vi "CRYReport Main.vi"() -> ()   [LabVIEW 2013]
uses:
  CRYReport Global.vi
  CRYWindow/DataView/SubVI/CRYData View Global.vi
  CRYSystem/Data/CRYData & result stacks global.vi
  CRYProject/CRYProject Editor Global.vi
  PrintTxDocDLL.dll
panel:
  in  "ADD_FRAME":bool
  in  "sViewType":string="DataView"
  in  "BtnDATE":bool
  in  "BtnSN":bool
  in  "BtnLot":bool
  in  "BtnOpen":bool
  in  "sInsertVIName":string
  in  "StateOut":bool
  in  "bChange":bool
  in  "BtnPageSize":bool
  in  "sPageSize":string
  in  "BtnPage":bool
  in  "Combo Box":string(combo)
  in  "BtnImage":bool
  in  "BtnPrint":bool
  in  "BtnSave":bool
  in  "TXButtonBar":refnum<k7>(container)
  in  "TXRuler":refnum<k7>(container)
  in  "TXTextControl":refnum<k7>(container)
  in  "stop":bool
  in  "TXStatusBar":refnum<k7>(container)
  in  "bPrintStatus":bool
  in  "bPageStatus":bool
  in  "bStateLoad":bool
  in  "bHitVIS":bool
  in  "InsertVI":bool
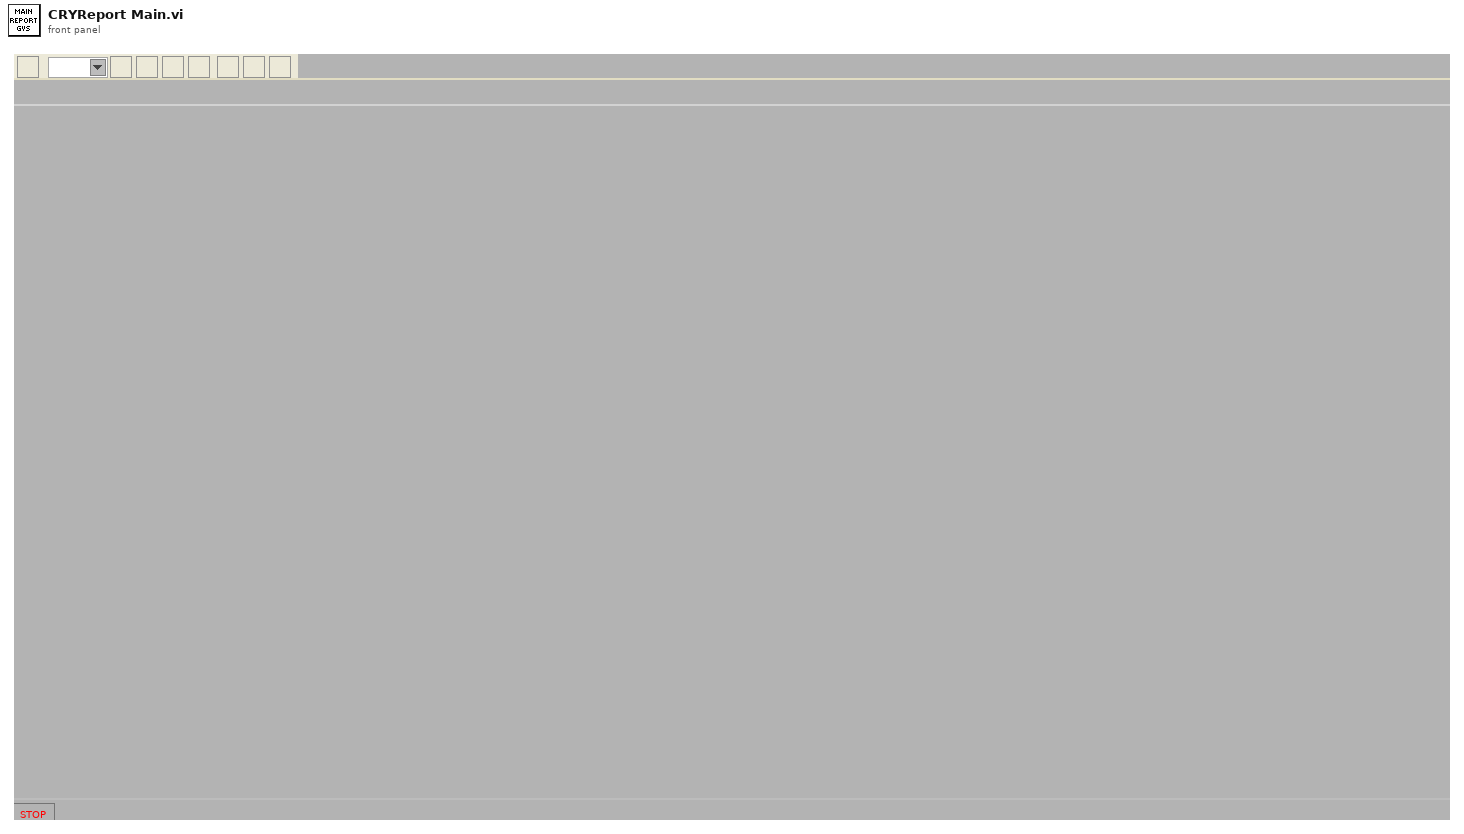
[diagram p1: front panel]
types:
  T1 = cluster{"sAction":string, "sType":string, "sQueueName":string, "sGraphName":string, "sData":string, "nData":i32, "pVIRef":refnum<vi>, "pSPRef":refnum<vi>}
  T2 = enum16{"Left Button", "Center Button", "Right Button", "Window Close"}
  T3 = enum16{"OK", "Yes", "YesNo", "YesNoCancel", "ReplaceAppend"}
  T4 = typedef "CRYDrag Graph.ctl" = cluster{"GraphType":string, "GraphData":variant}
  T5 = typedef "CRYTS.ctl" = cluster{"No.TS":u16, "TS File Path":path, "TS Name":string, "EditStepName":string, "Steps":T6[], "New State":bool, "Change State":bool, "Flattened CurveLib Data":string, "Document Data":string, "EditStepNo":u16, "Operator Start File":string, "Sequence Type":string, "Sequence Language":string}
  T6 = typedef "CRYStep.ctl" = cluster{"No.VI":i32, "Category":string, "StepName":string, "Seq setup flattened":string, "Comment":string, "Steps config.":bool[], "Jump config":i32[], "Start":dbl, "Increment":dbl, "Name":string, "Unit":string, "Y data":u16, "Y prefix":string, "Y dB ref":dbl, "Y unit":string, "Repeat State Array":cluster{"Start":dbl, "Increment":dbl, "Count":i32, "Num":i32}[]}
  T7 = cluster{"nCount":i16, "cFrameList":cluster{"nID":i16, "sName":string, "pVIRef":refnum<vi>, "pSPRef":refnum<vi>, "sTitle":string, "nIDObject":i16, "nIDV":i16, "nWidth":i16, "nHeight":i16, "bImgChange":bool, "sType":string, "sState":string, "sPosition":string, "sData":string}[], "sData":string}
  T8 = cluster{"nID":i16, "sName":string, "pVIRef":refnum<vi>, "pSPRef":refnum<vi>, "sTitle":string, "nIDObject":i16, "nIDV":i16, "nWidth":i16, "nHeight":i16, "bImgChange":bool, "sType":string, "sState":string, "sPosition":string, "sData":string}[]
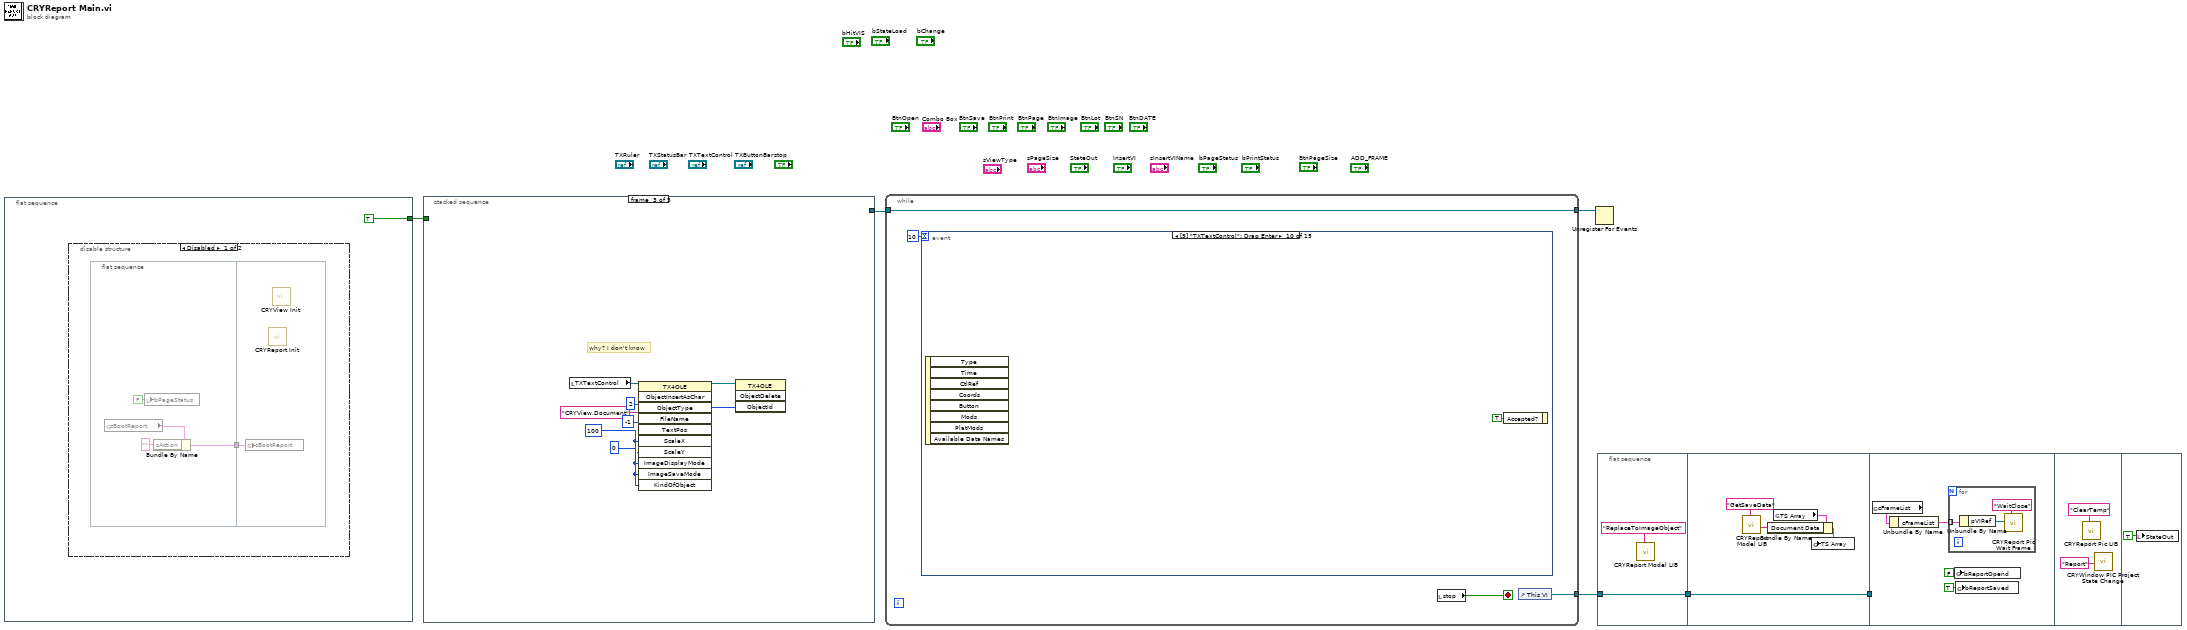
[diagram p0: block diagram]
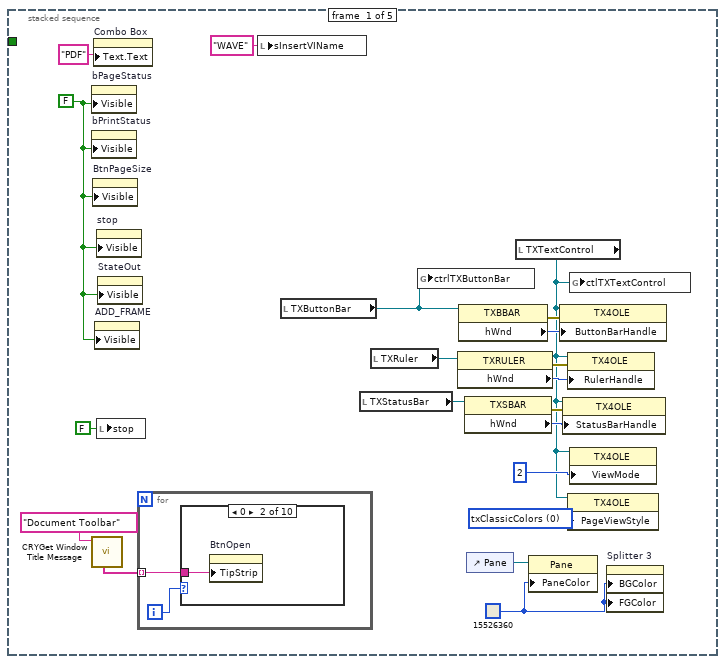
[diagram p3: hidden frame]
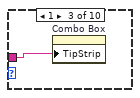
[diagram p5: hidden frame]
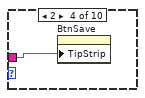
[diagram p6: hidden frame]
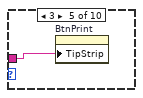
[diagram p7: hidden frame]
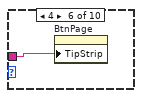
[diagram p8: hidden frame]
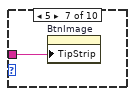
[diagram p9: hidden frame]
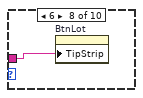
[diagram p10: hidden frame]
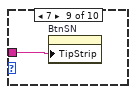
[diagram p11: hidden frame]
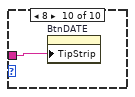
[diagram p12: hidden frame]
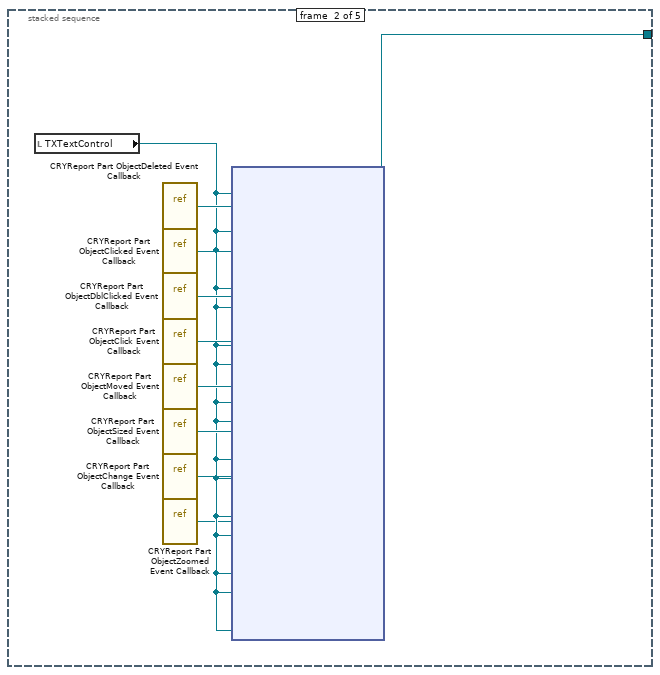
[diagram p13: hidden frame]
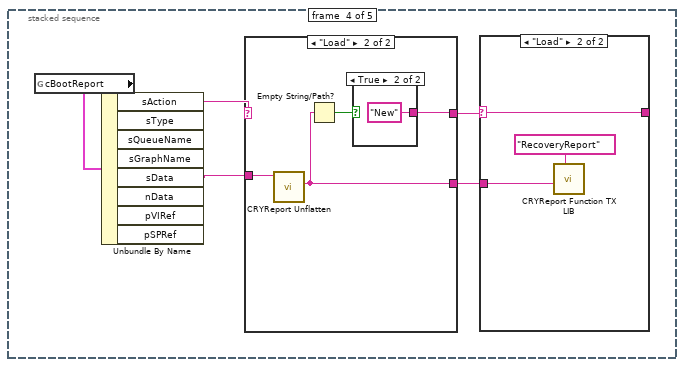
[diagram p14: hidden frame]
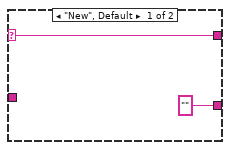
[diagram p16: hidden frame]
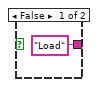
[diagram p17: hidden frame]
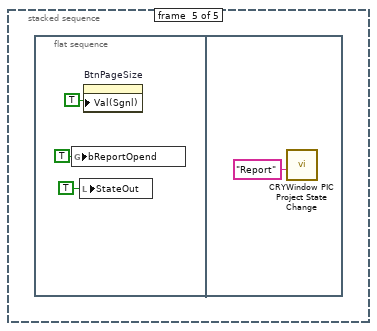
[diagram p18: hidden frame]
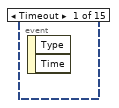
[diagram p19: hidden frame]
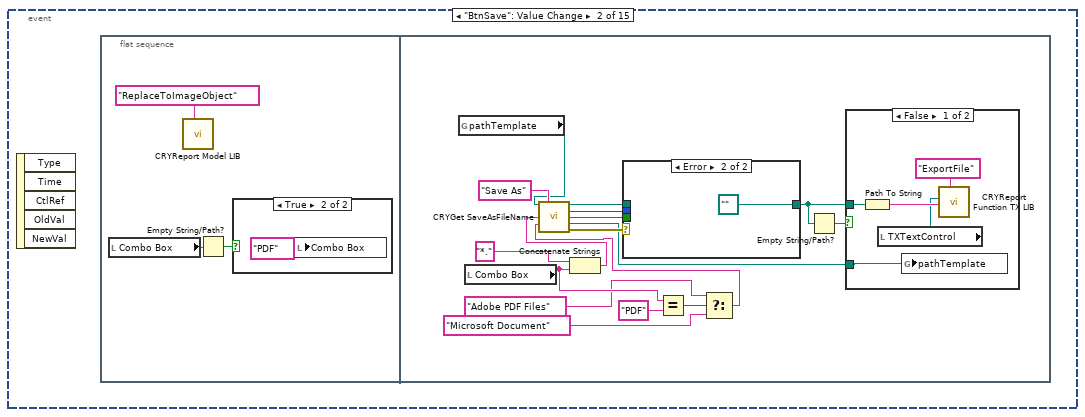
[diagram p20: hidden frame]
diagram:
  n1 = flat-sequence {
    tunnel: [TRUE] -> w3
    frame #0 {
      n2 = disable-structure shown="Disabled" {
        frame Disabled {
          n3 = flat-sequence {
            tunnel: [w9] -> w8
            tunnel: w8 -> [w13]
            frame #0 {
              n4 = global read "CRYReport Global.vi" "cBootReport"() -> (w11:T1)
              n5 = local write "bPageStatus"(FALSE ("bPageStatus")) -> ()
              n6 = Bundle By Name(cluster=w11, "sAction"="") -> (w9:T1)
            }
            frame #1 {
              n7 = global write "CRYReport Global.vi" "cBootReport"(w13) -> ()
              n8 = call "CRYReport Init.vi"() -> ()  [unwired: 12 in]
              n9 = call "CRYView Init.vi"() -> ()  [unwired: 12 in]
            }
          }
        }
        frame Enabled {
        }
      }
    }
  }
  n10 = stacked-sequence {
    tunnel: [_ w45 _ _ _] -> w6
    tunnel: w3 -> [_ _ _ _ _]
    frame #0 {
      w14 = FALSE ("Visible")
      w25 = u32 15526360
      w27 = 0 items=["txClassicColors", "txGradientColors"] ("PageViewStyle")
      n11 = property on="bPageStatus" class="Bool (strict)"("Visible"=w14) -> ()  [unwired: 2 in, 2 out]
      n12 = property on="bPrintStatus" class="Bool (strict)"("Visible"=w14) -> ()  [unwired: 2 in, 2 out]
      n13 = call "CRYGet Window Title Message.vi"("Kind"="Document Toolbar") -> ("Tip Strip"=w15:string[])  [unwired: 5 in, 5 out]
      n14 = property on="BtnPageSize" class="Bool (strict)"("Visible"=w14) -> ()  [unwired: 2 in, 2 out]
      n15 = property on="Combo Box" class="CmbBox"("Text.Text"="PDF") -> ()  [unwired: 2 in, 2 out]
      n16 = property on="ADD_FRAME" class="Bool (strict)"("Visible"=w14) -> ()  [unwired: 2 in, 2 out]
      n17 = property on="stop" class="Bool (strict)"("Visible"=w14) -> ()  [unwired: 2 in, 2 out]
      n18 = local write "stop"(FALSE ("stop")) -> ()
      n19 = property on="StateOut" class="Bool (strict)"("Visible"=w14) -> ()  [unwired: 2 in, 2 out]
      n20 = for {
        tunnel: w15 -> [w35] mode=indexing
        i -> [w34]
        n21 = case shown="0" w34 {
          tunnel: w35 -> [_ w36 w37 w38 w39 w40 w41 w42 w43 w44]
          frame Default {
          }
          frame 0 {
            n22 = property on="BtnOpen" class="Bool (strict)"("TipStrip"=w36) -> ()  [unwired: 2 in, 2 out]
          }
          frame 1 {
            n23 = property on="Combo Box" class="CmbBox"("TipStrip"=w37) -> ()  [unwired: 2 in, 2 out]
          }
          frame 2 {
            n24 = property on="BtnSave" class="Bool (strict)"("TipStrip"=w38) -> ()  [unwired: 2 in, 2 out]
          }
          frame 3 {
            n25 = property on="BtnPrint" class="Bool (strict)"("TipStrip"=w39) -> ()  [unwired: 2 in, 2 out]
          }
          frame 4 {
            n26 = property on="BtnPage" class="Bool (strict)"("TipStrip"=w40) -> ()  [unwired: 2 in, 2 out]
          }
          frame 5 {
            n27 = property on="BtnImage" class="Bool (strict)"("TipStrip"=w41) -> ()  [unwired: 2 in, 2 out]
          }
          frame 6 {
            n28 = property on="BtnLot" class="Bool (strict)"("TipStrip"=w42) -> ()  [unwired: 2 in, 2 out]
          }
          frame 7 {
            n29 = property on="BtnSN" class="Bool (strict)"("TipStrip"=w43) -> ()  [unwired: 2 in, 2 out]
          }
          frame 8 {
            n30 = property on="BtnDATE" class="Bool (strict)"("TipStrip"=w44) -> ()  [unwired: 2 in, 2 out]
          }
        }
      }
      n31 = local write "sInsertVIName"("WAVE" ("sData")) -> ()
      n32 = local read "TXButtonBar"() -> (w17:refnum<k7>)
      n33 = local read "TXStatusBar"() -> (w21:refnum<k7>)
      n34 = local read "TXRuler"() -> (w30:refnum<k7>)
      n35 = global write "CRYReport Global.vi" "ctrlTXButtonBar"(w17) -> ()
      n36 = property class="TXRULER"(reference=w30) -> (error out=w29:errorcluster, "hWnd"=w31:i32)  [unwired: 1 in, 1 out]
      n37 = property class="TXBBAR"(reference=w17) -> (error out=w33:errorcluster, "hWnd"=w32:i32)  [unwired: 1 in, 1 out]
      n38 = property class="TXSBAR"(reference=w21) -> (error out=w22:errorcluster, "hWnd"=w23:i32)  [unwired: 1 in, 1 out]
      n39 = control-ref of="Pane"() -> (w26:refnum<vi>)
      n40 = local read "TXTextControl"() -> (w19:refnum<k7>)
      n41 = property class="Pane"(reference=w26, "PaneColor"=w25) -> ()  [unwired: 1 in, 2 out]
      n42 = property class="TX4OLE"(reference=w19, error in=w33, "ButtonBarHandle"=w32) -> ()  [unwired: 2 out]
      n43 = property class="TX4OLE"(reference=w19, error in=w22, "StatusBarHandle"=w23) -> ()  [unwired: 2 out]
      n44 = property class="TX4OLE"(reference=w19, error in=w29, "RulerHandle"=w31) -> ()  [unwired: 2 out]
      n45 = property class="TX4OLE"(reference=w19, "PageViewStyle"=w27) -> ()  [unwired: 1 in, 2 out]
      n46 = global write "CRYReport Global.vi" "ctlTXTextControl"(w19) -> ()
      n47 = property class="TX4OLE"(reference=w19, "ViewMode"=i16 2) -> ()  [unwired: 1 in, 2 out]
      n48 = property on="Splitter 3" class="Splitter"("BGColor"=w25, "FGColor"=w25) -> ()  [unwired: 2 in, 2 out]
    }
    frame #1 {
      n49 = local read "TXTextControl"() -> (w47:refnum<k7>)
      n50 = vi-ref "CRYReport Part ObjectDeleted Event Callback.vi"() -> ("vi reference"=w54:refnum<vi>)
      n51 = vi-ref "CRYReport Part ObjectClicked Event Callback.vi"() -> ("vi reference"=w52:refnum<vi>)
      n52 = vi-ref "CRYReport Part ObjectDblClicked Event Callback.vi"() -> ("vi reference"=w53:refnum<vi>)
      n53 = vi-ref "CRYReport Part ObjectClick Event Callback.vi"() -> ("vi reference"=w51:refnum<vi>)
      n54 = vi-ref "CRYReport Part ObjectMoved Event Callback.vi"() -> ("vi reference"=w50:refnum<vi>)
      n55 = vi-ref "CRYReport Part ObjectSized Event Callback.vi"() -> ("vi reference"=w49:refnum<vi>)
      n56 = vi-ref "CRYReport Part ObjectChange Event Callback.vi"() -> ("vi reference"=w48:refnum<vi>)
      n57 = vi-ref "CRYReport Part ObjectZoomed Event Callback.vi"() -> ("vi reference"=w46:refnum<vi>)
      n58 = node(w47, w54, w47, w47, w52, w47, w47, w53, w47, w47, w51, w47, w47, w50, w47, w47, w49, w47, w47, w48, w47, w47, w46, w47) -> (w45:refnum<k27>)  [unwired: 2 in, 1 out]
    }
    frame #2 {
      w62 = i16 0 ("ImageDisplayMode")
      w59 = i16 100 ("ScaleX")
      # "why? I don't know"
      n59 = local read "TXTextControl"() -> (w55:refnum<k7>)
      n60 = invoke class="TX4OLE" method="ObjectInsertAsChar"(reference=w55, "ObjectType"=2, "FileName"="CRYView.Document", "TextPos"=-1, "ScaleX"=w59, "ScaleY"=w59, "ImageDisplayMode"=w62, "ImageSaveMode"=w62, "KindOfObject"=w62) -> (reference out=w60:refnum<k7>, "ObjectInsertAsChar"=w61:i16)  [unwired: 2 in, 9 out]
      n61 = invoke class="TX4OLE" method="ObjectDelete"(reference=w60, "ObjectId"=w61) -> ()  [unwired: 2 in, 4 out]
    }
    frame #3 {
      n62 = global read "CRYReport Global.vi" "cBootReport"() -> (w67:T1)
      n63 = Unbundle By Name(w67) -> ("sAction"=w66:string, "sData"=w65:string)  [unwired: 6 out]
      n64 = case shown="\"Load\"" w66 {
        selector: w66 -> [w73 _]
        tunnel: [w73 w75] -> w64
        tunnel: w65 -> [_ w77]
        tunnel: ["" ("Checked Flatten Report") w74] -> w63
        frame "New", Default {
        }
        frame "Load" {
          n65 = call "CRYReport Unflatten.vi"("Flatten Report"=w77) -> ("Checked Flatten Report"=w74:string)  [unwired: 8 in, 2 out]
          n66 = Empty String/Path?(string/path=w74) -> (empty?=w76:bool)
          n67 = case shown="True" w76 {
            tunnel: ["Load" "New"] -> w75
            frame False {
            }
            frame True {
            }
          }
        }
      }
      n68 = case shown="\"Load\"" w64 {
        selector: w64 -> [w68 w71]
        tunnel: [w68 w71] -> _
        tunnel: w63 -> [_ w69]
        frame "New", Default {
        }
        frame "Load" {
          n69 = call "CRYReport Function TX LIB.vi"("sAction"="RecoveryReport", "sData"=w69) -> ()  [unwired: 7 in, 3 out]
        }
      }
    }
    frame #4 {
      n70 = flat-sequence {
        frame #0 {
          n71 = global write "CRYReport Global.vi" "bReportOpend"(TRUE ("bPreportOpend")) -> ()
          n72 = local write "StateOut"(TRUE ("StateOut")) -> ()
          n73 = property on="BtnPageSize" class="Bool (strict)"("Val(Sgnl)"=TRUE ("BtnPageSize")) -> ()  [unwired: 2 in, 2 out]
        }
        frame #1 {
          n74 = call "CRYWindow PIC Project State Change.vi"("sData"="Report") -> ()  [unwired: 11 in]
        }
      }
    }
  }
  n75 = while {
    tunnel: [w87] -> w4
    tunnel: w6 -> [w86]
    tunnel: [w86] -> w5
    stop <- w84 stop-if-true
    n76 = event shown="[9] \"TXTextControl\": Drag Enter" {
      selector: _ -> [_ _ _ _ _ _ _ _ _ _ _ _ _ _ _]
      dyn-events: _ -> [_ _ _ _ _ _ _ _ _ _ _ _ _ _ _]
      timeout: 10 -> [_ _ _ _ _ _ _ _ _ _ _ _ _ _ _]
      event Timeout {
        n77 = event-data() -> ()  [unwired: 1 in, 2 out]
      }
      event "BtnSave": Value Change {
        n78 = event-data() -> ()  [unwired: 1 in, 5 out]
        n79 = flat-sequence {
          frame #0 {
            n80 = local read "Combo Box"() -> (w89:string)
            n81 = call "CRYReport Model LIB.vi"("sAction"="ReplaceToImageObject") -> ()  [unwired: 9 in, 2 out]
            n82 = Empty String/Path?(string/path=w89) -> (empty?=w88:bool)
            n83 = case shown="True" w88 {
              frame False {
              }
              frame True {
                n84 = local write "Combo Box"("PDF" ("Combo Box")) -> ()
              }
            }
          }
          frame #1 {
            n85 = global read "CRYReport Global.vi" "pathTemplate"() -> (w99:path)
            n86 = local read "Combo Box"() -> (w97:string)
            n87 = Concatenate Strings("*." ("string"), w97) -> (w107:string)
            n88 = Equal?(x=w97, y="PDF") -> (x = y?=w95:bool)
            n89 = Select(t="Adobe PDF Files" ("pattern label"), s=w95, f="Microsoft Document" ("pattern label")) -> (s? t:f=w93:string)
            n90 = call "CRYGet SaveAsFileName.vi"("Start path"=w99, "TitleName"="Save As", "pattern (all files)"=w107, "pattern label"=w93) -> ("Path"=w108:path, "Which Button?"=w104:T2, "Is Replace?"=w105:bool, "stripped path"=w98:path, "error out"=w103:errorcluster)  [unwired: 5 in, 2 out]
            n91 = case shown="Error" w103 {
              tunnel: w108 -> [w118 _]
              tunnel: w104 -> [w117 _]
              tunnel: w105 -> [w119 _]
              tunnel: [w114 path "" ("Path")] -> w101
              frame No Error {
                n92 = case shown="True" w119 {
                  tunnel: w118 -> [w122 w124]
                  tunnel: [w122 w124] -> w115
                  tunnel: w117 -> [w123 w125]
                  tunnel: [w123 w125] -> w116
                  frame False {
                  }
                  frame True {
                  }
                }
                n93 = case shown="\"Left Button\", Default" w116 {
                  tunnel: w115 -> [w120 _]
                  tunnel: [w120 path "" ("Path")] -> w114
                  frame "Left Button", Default {
                  }
                  frame "Center Button" {
                  }
                }
              }
              frame Error {
              }
            }
            n94 = Empty String/Path?(string/path=w101) -> (empty?=w100:bool)
            n95 = case shown="False" w100 {
              tunnel: w101 -> [w113 _]
              tunnel: w98 -> [w109 _]
              frame False {
                n96 = Path To String(path=w113) -> (string=w112:string)
                n97 = local read "TXTextControl"() -> (w110:refnum<k7>)
                n98 = global write "CRYReport Global.vi" "pathTemplate"(w109) -> ()
                n99 = call "CRYReport Function TX LIB.vi"("sAction"="ExportFile", "sData"=w112, "TXTextControl"=w110) -> ()  [unwired: 6 in, 3 out]
              }
              frame True {
              }
            }
          }
        }
      }
      event "BtnPageSize": Value Change {
        w139 = 0.5 ("y")
        w142 = 25.4 ("y")
        w145 = 1440.0 ("y")
        n100 = event-data() -> ()  [unwired: 1 in, 5 out]
        n101 = local read "TXTextControl"() -> (w127:refnum<k7>)
        n102 = property class="TX4OLE"(reference=w127) -> ("PageWidth"=w147:i32)  [unwired: 1 in, 2 out]
        n103 = property class="TX4OLE"(reference=w127) -> ("PageHeight"=w146:i32)  [unwired: 1 in, 2 out]
        n104 = Divide(x=w147, y=w145) -> (x/y=w144:dbl)
        n105 = Divide(x=w146, y=w145) -> (x/y=w143:dbl)
        n106 = Multiply(x=w143, y=w142) -> (x*y=w140:dbl)
        n107 = Multiply(x=w144, y=w142) -> (x*y=w141:dbl)
        n108 = Add(x=w141, y=w139) -> (x+y=w136:dbl)
        n109 = Add(x=w140, y=w139) -> (x+y=w135:dbl)
        n110 = Number To Decimal String(number=w136) -> (decimal integer string=w138:string)  [unwired: 1 in]
        n111 = Number To Decimal String(number=w135) -> (decimal integer string=w134:string)  [unwired: 1 in]
        n112 = Concatenate Strings(w138, "*" ("string"), w134) -> (w129:string)
        n113 = case shown="\"148*210\", \"210*148\"" w129 {
          tunnel: ["Custom" "A4" "A3" "A5" "B4" "B5" "Postcard" "Legal" "Tabloid" "Executive" "Screen" "Letter" "Letter Extra" "Letter Plus" "Qurato" "Statement" "SuperA" "SuperB"] -> w131
          frame Default {
          }
          frame "210*297", "297*210" {
          }
          frame "297*420", "420*297" {
          }
          frame "148*210", "210*148" {
          }
          frame "257*364", "364*257" {
          }
          frame "182*257", "257*182" {
          }
          frame "100*147", "147*100" {
          }
          frame "216*356", "356*216" {
          }
          frame "280*432", "432*280" {
          }
          frame "185*267", "267*185" {
          }
          frame "132*166", "166*132" {
          }
          frame "216*280", "280*216" {
          }
          frame "242*305", "305*242" {
          }
          frame "216*323", "323*216" {
          }
          frame "215*275", "275*215" {
          }
          frame "140*216", "216*140" {
          }
          frame "227*356", "356*227" {
          }
          frame "305*487", "487*305" {
          }
        }
        n114 = Concatenate Strings(w131, "(" ("string"), w129, ")" ("string"), "mm" ("string")) -> (w128:string)
        n115 = local write "sPageSize"(w128) -> ()
      }
      event "BtnOpen": Value Change {
        n116 = event-data() -> ()  [unwired: 1 in, 5 out]
        n117 = local read "TXTextControl"() -> (w169:refnum<k7>)
        n118 = invoke class="TX4OLE" method="GetLineCount"(reference=w169) -> ("GetLineCount"=w168:i32)  [unwired: 2 in, 2 out]
        n119 = Greater Than 0?(x=w168) -> ()  [unwired: 1 out]
        n120 = case shown="False" FALSE {
          tunnel: [T2."Left Button" ("Which Button?") w171] -> w167
          frame False {
          }
          frame True {
            n121 = call <vilib>:"Three Button Dialog.vi"("message"="Do you want replace document ?") -> ("Which Button?"=w171:T2)  [unwired: 10 in]
          }
        }
        n122 = case shown="\"Left Button\"" w167 {
          frame "Left Button" {
            n123 = flat-sequence {
              frame #0 {
                n124 = call "CRYReport Model LIB.vi"("sAction"="ReplaceToImageObject") -> ()  [unwired: 9 in, 2 out]
              }
              frame #1 {
                n125 = global read "CRYReport Global.vi" "pathTemplate"() -> (w176:path)
                n126 = call "CRYGet LoadFileName.vi"("pattern label"="Microsoft Document", "pattern (all files)"="*.doc" ("string"), "TitleName"="Open As", "Category Name"="doc" ("string"), "Start path"=w176) -> ("error out"=w180:errorcluster, "stripped path"=w175:path, "Which Button?"=w181:T2, "Path"=w182:path)  [unwired: 3 in]
                n127 = case shown="No Error" w180 {
                  tunnel: w182 -> [w184 _]
                  tunnel: w181 -> [w185 _]
                  tunnel: w175 -> [w183 _]
                  frame No Error {
                    n128 = case shown="\"Center Button\", Default" w185 {
                      tunnel: w184 -> [w190 _]
                      tunnel: w183 -> [w186 _]
                      frame "Left Button" {
                        n129 = Path To String(path=w190) -> (string=w189:string)
                        n130 = local read "TXTextControl"() -> (w187:refnum<k7>)
                        n131 = global write "CRYReport Global.vi" "pathTemplate"(w186) -> ()
                        n132 = call "CRYReport Function TX LIB.vi"("sAction"="OpenFile", "sData"=w189, "TXTextControl"=w187) -> ()  [unwired: 6 in, 3 out]
                      }
                      frame "Center Button", Default {
                      }
                    }
                  }
                  frame Error {
                  }
                }
              }
            }
          }
          frame Default {
          }
        }
      }
      event "BtnImage": Value Change {
        n133 = event-data() -> ()  [unwired: 1 in, 5 out]
        n134 = call "File Dialog"("prompt"="Select a File to Open" ("TitleName"), "pattern (all files)"="*.bmp;*.jpg;*.png;*.tiff") -> ("selected path"=w198:path, "exists"=w197:bool, "error out"=w196:errorcluster)  [unwired: 5 in, 6 out]
        n135 = case shown="No Error" w196 {
          tunnel: w198 -> [w212 _]
          tunnel: w197 -> [w211 _]
          tunnel: [w213 path "" ("Path")] -> w193
          frame No Error {
            n136 = case shown="True" w211 {
              tunnel: w212 -> [w214 _]
              tunnel: [w214 path "" ("Path")] -> w213
              frame True {
              }
              frame False {
              }
            }
          }
          frame Error {
          }
        }
        n137 = Path To String(path=w193) -> (string=w191:string)
        n138 = Empty String/Path?(string/path=w191) -> (empty?=w192:bool)
        n139 = case shown="False" w192 {
          tunnel: w191 -> [w201 _]
          tunnel: w193 -> [w200 _]
          frame False {
            n140 = call <vilib>:"Get File Extension.vi"("file"=w200) -> ("lowercase file extension"=w199:string)  [unwired: 7 in, 3 out]
            n141 = case shown="\"False\", Default" w199 {
              tunnel: w201 -> [_ w207]
              frame "False", Default {
                n142 = call "CRYGet Error Message.vi"("Error No"=0, "Kind"="Document") -> ("Message"=w203:string, "Window Title"=w202:string)  [unwired: 4 in, 4 out]
                n143 = call "CRYMessage Dialog.vi"("Window Title"=w202, "YesNoCancel"=T3."OK", "Message Content"=w203) -> ()  [unwired: 7 in, 2 out]
              }
              frame "bmp", "jpg", "png", "tiff" {
                w208 = i16 100 ("ScaleX")
                n144 = local read "TXTextControl"() -> (w210:refnum<k7>)
                n145 = invoke class="TX4OLE" method="ImageInsertAsChar"(reference=w210, "FileName"=w207, "TextPos"=-1, "ScaleX"=w208, "ScaleY"=w208) -> ()  [unwired: 2 in, 7 out]
              }
            }
          }
          frame True {
          }
        }
      }
      event Pane Size {
        n146 = event-data() -> ()  [unwired: 1 in, 5 out]
        n147 = control-ref of="Splitter 3"() -> (w218:refnum<vi>)
        n148 = property class="Splitter"(reference=w218, "Position"=280 ("Splitter Position")) -> (error out=w217:errorcluster)  [unwired: 1 in, 1 out]
        n149 = case shown="No Error" w217 {
          frame No Error {
          }
          frame Error {
          }
        }
      }
      event "BtnPrint": Value Change {
        n150 = event-data() -> ()  [unwired: 1 in, 5 out]
        n151 = flat-sequence {
          frame #0 {
            n152 = call "CRYReport Model LIB.vi"("sAction"="ReplaceToImageObject") -> ()  [unwired: 9 in, 2 out]
          }
          frame #1 {
            n153 = global read "CRYReport Global.vi" "pathTemp"() -> (w223:path)
            n154 = Build Path(base path=w223, name or relative path="PRINT.txw" ("name")) -> (appended path=w226:path)
            n155 = local read "TXTextControl"() -> (w224:refnum<k7>)
            n156 = Path To String(path=w226) -> (string=w225:string)
            n157 = Strip Path(path=w223) -> (stripped path=w222:path)  [unwired: 1 out]
            n158 = Path To String(path=w222) -> (string=w221:string)
            n159 = invoke class="TX4OLE" method="Save"(reference=w224, "FileName"=w225, "Offset"=0, "Format"=8, "CurSelection"=FALSE) -> ("FileName"=w228:string)  [unwired: 2 in, 6 out]
            n160 = dll-call lib="D:/A_CRYSoundLab_Work/CRY6181/CRYDocument/PrintTxDocDLL.dll" fn="PrintGVSDoc"("szPath"=w221, "szFileName"=w228) -> ()  [unwired: 3 in, 5 out]
          }
        }
      }
      event "InsertVI": Value Change {
        n161 = event-data() -> ()  [unwired: 1 in, 5 out]
        n162 = local read "TXTextControl"() -> (w232:refnum<k7>)
        n163 = local read "sInsertVIName"() -> (w233:string)
        n164 = call "CRYReport Function TX LIB.vi"("sAction"="NewFrame", "sData"=w233, "TXTextControl"=w232) -> ()  [unwired: 6 in, 3 out]
      }
      event "ADD_FRAME": Value Change {
        n165 = event-data() -> ()  [unwired: 1 in, 5 out]
        n166 = flat-sequence {
          frame #0 {
            n167 = call "CRYReport Model LIB.vi"("sAction"="ReplaceToImageObject") -> ()  [unwired: 9 in, 2 out]
          }
          frame #1 {
            n168 = local read "sInsertVIName"() -> (w237:string)
            n169 = local read "TXTextControl"() -> (w236:refnum<k7>)
            n170 = call "CRYReport Function TX LIB.vi"("sAction"="AddNewFrame", "sData"=w237, "TXTextControl"=w236) -> ()  [unwired: 6 in, 3 out]
          }
        }
      }
      event "TXTextControl": Drag Enter {
        n171 = event-data() -> ()  [unwired: 1 in, 8 out]
        n172 = event-data("Accepted?"=TRUE) -> ()  [unwired: 1 in, 1 out]
      }
      event "TXTextControl": Drop {
        n173 = event-data() -> ()  [unwired: 1 in, 8 out]
        n174 = flat-sequence {
          tunnel: [TRUE] -> w240
          frame #0 {
            n175 = call "CRYReport Model LIB.vi"("sAction"="ReplaceToImageObject") -> ()  [unwired: 9 in, 2 out]
          }
          frame #1 {
            n176 = global read "CRYData View Global.vi" "Drag into Graph"() -> (w243:T4)
            n177 = Unbundle By Name(w243) -> ("GraphType"=w242:string)
            n178 = flat-sequence {
              tunnel: w242 -> [w246]
              tunnel: w243 -> [w245]
              frame #0 {
                n179 = local write "sInsertVIName"(w246) -> ()
                n180 = global write "CRYReport Global.vi" "cDropData"(w245) -> ()
              }
              frame #1 {
                n181 = property on="InsertVI" class="Bool (strict)"("Val(Sgnl)"=TRUE ("Value (Signaling)")) -> ()  [unwired: 2 in, 2 out]
              }
            }
          }
        }
        n182 = event-data("Accepted?"=w240) -> ()  [unwired: 1 in, 1 out]
      }
      event "BtnPage": Value Change {
        n183 = event-data() -> ()  [unwired: 1 in, 5 out]
        n184 = flat-sequence {
          tunnel: [w249] -> w248
          tunnel: w248 -> [w251]
          frame #0 {
            n185 = local read "TXTextControl"() -> (w249:refnum<k7>)
            n186 = call "CRYReport Model LIB.vi"("sAction"="ReplaceToImageObject") -> ()  [unwired: 9 in, 2 out]
          }
          frame #1 {
            n187 = invoke class="TX4OLE" method="SectionFormatDialog"(reference=w251, "ActiveTab"=i16 0) -> ("SectionFormatDialog"=w252:bool)  [unwired: 2 in, 3 out]
            n188 = case shown="True" w252 {
              frame False {
              }
              frame True {
                n189 = property on="BtnPageSize" class="Bool (strict)"("Val(Sgnl)"=FALSE ("Value (Signaling)")) -> ()  [unwired: 2 in, 2 out]
              }
            }
          }
        }
      }
      event "BtnLot": Value Change {
        n190 = event-data() -> ()  [unwired: 1 in, 5 out]
        n191 = local read "TXTextControl"() -> (w255:refnum<k7>)
        n192 = global read "CRYData & result stacks global.vi" "Lot #"() -> (w256:string)
        n193 = call "CRYReport Pic Insert Text.vi"("sData"=w256, "TXTextControl"=w255) -> ()  [unwired: 10 in]
      }
      event "BtnSN": Value Change {
        n194 = event-data() -> ()  [unwired: 1 in, 5 out]
        n195 = local read "TXTextControl"() -> (w257:refnum<k7>)
        n196 = global read "CRYData & result stacks global.vi" "Serial #"() -> (w258:string)
        n197 = call "CRYReport Pic Insert Text.vi"("sData"=w258, "TXTextControl"=w257) -> ()  [unwired: 10 in]
      }
      event "BtnDATE": Value Change {
        n198 = event-data() -> ()  [unwired: 1 in, 5 out]
        n199 = local read "TXTextControl"() -> (w259:refnum<k7>)
        n200 = Get Date/Time String(date format (0)=enum16{"short", "long", "abbreviated"}."short", want seconds? (F)=TRUE) -> (date string=w262:string, time string=w261:string)  [unwired: 1 in]
        n201 = Format Into String(format string="%s %s", w262, w261) -> (resulting string=w260:string)  [unwired: 2 in, 1 out]
        n202 = call "CRYReport Pic Insert Text.vi"("sData"=w260, "TXTextControl"=w259) -> ()  [unwired: 10 in]
      }
    }
    n203 = local read "stop"() -> (w84:bool)
    n204 = control-ref of="This VI"() -> (w87:refnum<vi>)
  }
  n205 = Unregister For Events(event registration refnum=w5) -> ()  [unwired: 1 in, 1 out]
  n206 = flat-sequence {
    tunnel: w4 -> [w267]
    tunnel: [w267] -> w1
    tunnel: [w272] -> w2
    tunnel: w1 -> [w272]
    tunnel: w2 -> [_]
    frame #0 {
      n207 = call "CRYReport Model LIB.vi"("sAction"="ReplaceToImageObject") -> ()  [unwired: 9 in, 2 out]
    }
    frame #1 {
      n208 = call "CRYReport Model LIB.vi"("sAction"="GetSaveData") -> ("sData_Out"=w270:string)  [unwired: 9 in, 1 out]
      n209 = global read "CRYProject Editor Global.vi" "TS Array"() -> (w268:T5)
      n210 = Bundle By Name(cluster=w268, "Document Data"=w270) -> (w269:T5)
      n211 = global write "CRYProject Editor Global.vi" "TS Array"(w269) -> ()
    }
    frame #2 {
      n212 = global read "CRYReport Global.vi" "cFrameList"() -> (w276:T7)
      n213 = Unbundle By Name(w276) -> ("cFrameList"=w275:T8)
      n214 = for {
        tunnel: w275 -> [w278] mode=indexing
        n215 = Unbundle By Name(w278) -> ("pVIRef"=w277:refnum<vi>)
        n216 = call "CRYReport Pic Wait Frame.vi"("sAction"="WaitClose", "vi reference"=w277) -> ()  [unwired: 9 in, 1 out]
      }
      n217 = global write "CRYReport Global.vi" "bReportOpend"(FALSE ("bPreportOpend")) -> ()
      n218 = global write "CRYReport Global.vi" "bReportSaved"(TRUE ("bPreportOpend")) -> ()
    }
    frame #3 {
      n219 = call "CRYReport Pic LIB.vi"("sAction"="ClearTemp") -> ()  [unwired: 7 in, 4 out]
      n220 = call "CRYWindow PIC Project State Change.vi"("sData"="Report") -> ()  [unwired: 11 in]
    }
    frame #4 {
      n221 = local write "StateOut"(TRUE ("StateOut")) -> ()
    }
  }
